vi "CSM - Destroy Global Log Event.vi"(6 "Timeout In ms (5000ms)":i32=5000, 8 "Error In":errorcluster caption="error in (no error)", 9 "Force Destroy? (F)":bool, 11 "CSM Global Log Event":refnum<user-event>) -> (0 "error out":errorcluster)   [LabVIEW 2017, in "Communicable State Machine.lvlib"]
doc: "Releases the CSM global log user event refnum.\n\n\n> [!NOTE] <b>CSM Global Log Functionality</b>\n>\n> The CSM Global Log functionality is used to view global log change events, serving scenarios such as debugging and monitoring.\n> The following is the information that can be logged:\n> - Module state modifications\n> - Inter-module message communication, including data returns\n> - Message completion records of asynchronous and synchronous messages, `AsyncMsg Complete` and `SyncMsg Complete`, which carry the response\n> - Module status publishing\n> - Module creation and destruction\n> - Module state registration and unregistration\n> - Error information handled by modules\n> - User-defined events\n>\n> Debugging tools are primarily developed based on the Global Log API. You can develop debugging tools according to your own needs.\n\n\n> [!NOTE] <b>CSM Global Log Acquisition Methods</b>\n>\n> CSM provides two methods for acquiring global logs: Queue and Event. The Queue processing method is recommended because the queue interface is more efficient and offers greater flexibility in selecting log processing schemes based on the number of accumulated logs in the queue.\n\n\n<b>Reference Examples</b>:\n- `4. Advance Examples\\Filter From Source(Event).vi`\n- `4. Advance Examples\\Filter From Subscriber(Event).vi`\n\n-- <b>Controls</b> --\n- <b>CSM Global Log Event</b>: CSM global log user event refnum.\n- <b>Force Destroy? (F)</b>: Whether to force destruction. The default is FALSE, which specifies not to force.\n- <b>Timeout In ms (5000ms)</b>: Timeout duration. The default is 5000 ms."
uses:
  Communicable State Machine.lvlib
  _Support/Typedef/_CSM_GlobalLog_MSG.ctl
  _Support/Typedef/_CSM_Response Source Message.ctl
  _Support/Typedef/_CSM_GlobalLog_MSG_TYPE.ctl
  _Support/ChangeFlag/ChangeFlag-Write.vi
  Utility/Random Change Flag.vi
  _Support/ChangeFlag/ChangeFlagDB.vi
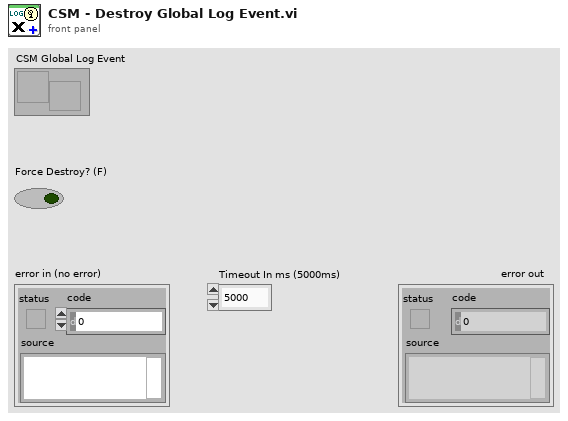
[diagram p1: front panel]
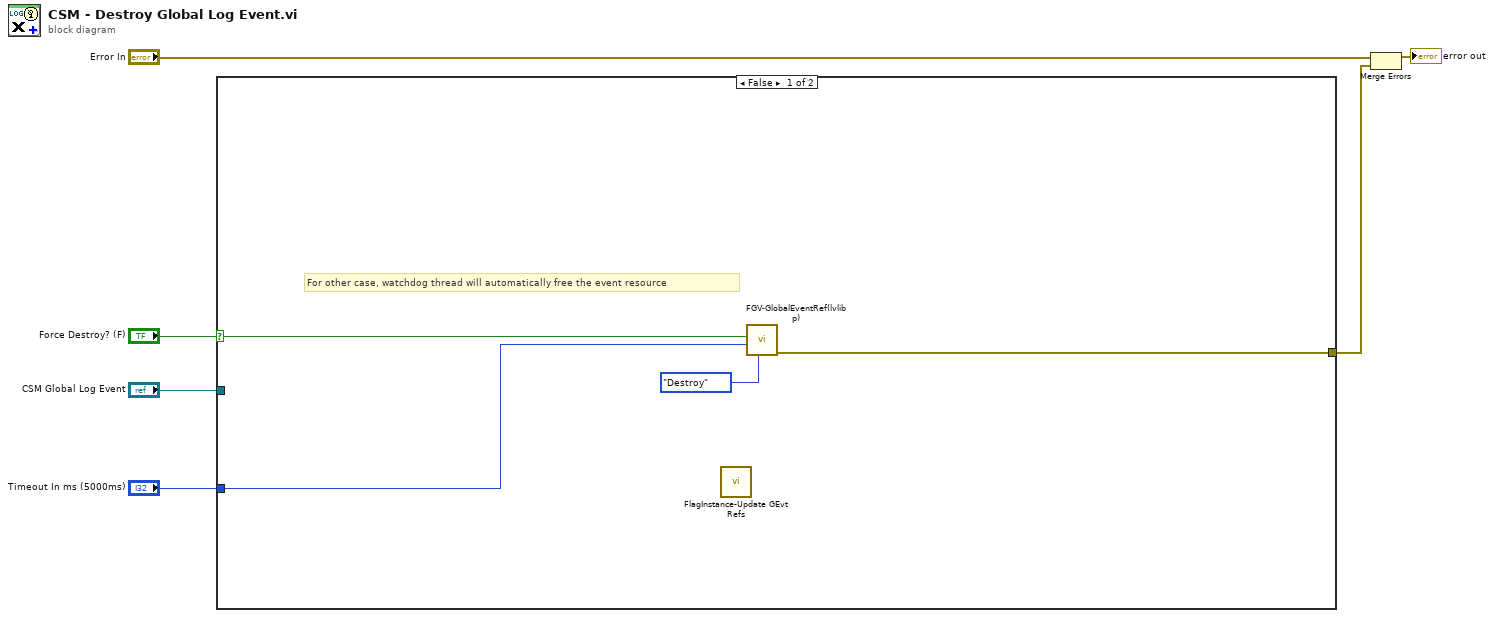
[diagram p0: block diagram]
diagram:
  n1 = case shown="False" "Force Destroy? (F)" {
    selector: "Force Destroy? (F)" -> [w10 _]
    tunnel: [w8 _] -> w4
    tunnel: "CSM Global Log Event" -> [_ _]
    tunnel: "Timeout In ms (5000ms)" -> [w9 _]
    frame False {
      # "For other case, watchdog thread will automatically free the event resource"
      n2 = call "FlagInstance-Update GEvt Refs.vi"() -> ()  [unwired: 10 in, 2 out]
      n3 = call "FGV-GlobalEventRef(lvlibp).vi"("Operation"=enum16{"Create", "Read", "Destroy"}."Destroy", "Timeout In ms (5000 ms)"=w9, "Force Destroy?"=w10) -> ("error out"=w8:errorcluster)  [unwired: 7 in, 1 out]
    }
    frame True {
    }
  }
  n4 = Merge Errors("Error In", w4) -> (→"error out":errorcluster)
